vi "Problem_Line_Constant.vi"() -> (3 "Problem Line":string="'/number of jobs, number of machines, time seed, machine seed, upper bound, lower bound :/'")   [LabVIEW 2013]
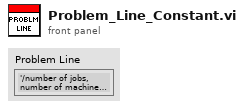
[diagram p1: front panel]
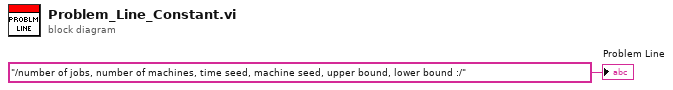
[diagram p0: block diagram]
diagram:
  "Problem Line" <- "/number of jobs, number of machines, time seed, machine seed, upper bound, lower bound :/" ("String")
